vi "Counter.vi"(1 "Reset?":bool, 2 "Increment?":bool, 3 "Increment Value":u32=1, 4 "Initial Value":u32) -> (0 "Value":u32)   [LabVIEW 2016]
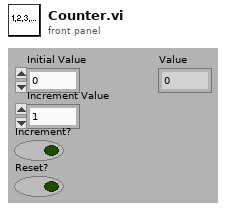
[diagram p1: front panel]
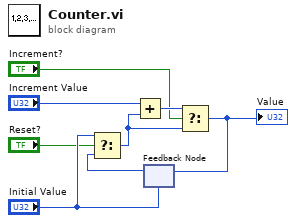
[diagram p0: block diagram]
diagram:
  n1 = feedback #1("Initial Value") -> (w2:u32)
  n2 = Select(t="Initial Value", s="Reset?", f=w2) -> (s? t:f=w4:u32)
  n3 = Add(x="Increment Value", y=w4) -> (x+y=w8:u32)
  n4 = Select(t=w8, s="Increment?", f=w4) -> (s? t:f=w7:u32)
  "Value" <- w7
  n5 = feedback-in #1(w7) -> ()
